vi "GaussianFit1D.vi"(0 "Cut":dbl[](graph)=[201.0, 170.0, 133.0, 114.0, 97.0, 133.0, 100.0, 5.0, 49.0, 50.0, 23.0, -22.0, -18.0, 16.0, 32.0, 1.0, -40.0, -42.0, -16.0, 11.0, -45.0, 12.0, -44.0, 20.0, -75.0, -48.0, 7.0, -12.0, -59.0, -11.0, -91.0, -34.0, -8.0, 3.0, -81.0, -7.0, -61.0, -16.0, -12.0, -87.0, -53.0, -14.0, -17.0, -15.0, -2.0, -87.0, -43.0, -62.0, -21.0, -22.0, -84.0, 12.0, -74.0, -15.0, -65.0, -10.0, 23.0, -6.0, 151.0, 386.0, 1054.0, 2361.0, 4328.0, 5745.0, 7056.0, 6029.0, 3889.0, 2158.0, 764.0, 178.0, -14.0, -30.0, 42.0, 60.0, -25.0, 8.0, -41.0, 24.0, -82.0, -31.0, 3.0, -2.0, 44.0, -60.0, -18.0, 0.0, 33.0, 26.0, -27.0, -29.0, -16.0, 19.0, 14.0, -10.0, -36.0, -47.0, -663.0, -28.0, -32.0, -7.0]) -> (1 "Sigma":dbl format="%.2f", 2 "x":dbl format="%.2f")   [LabVIEW 2009]
uses:
  <vilib>/gmath/NI_Gmath.lvlib
  <vilib>/Analysis/NI_AALBase.lvlib
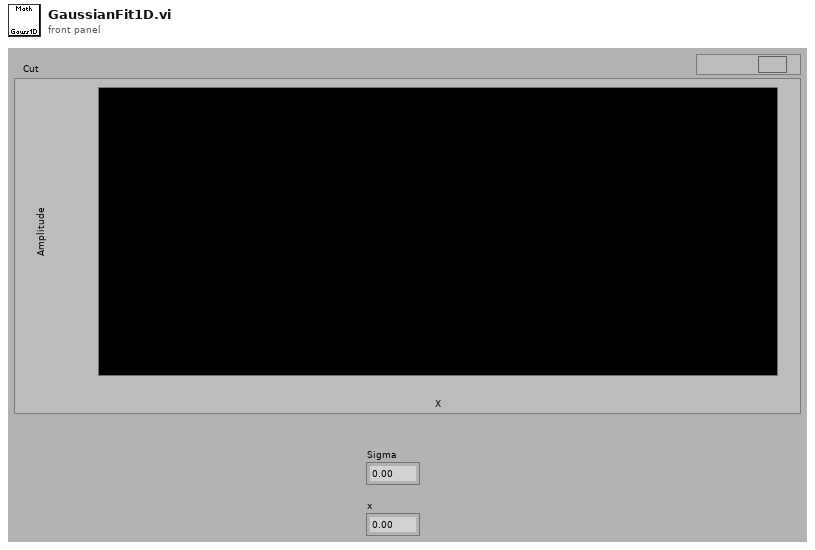
[diagram p1: front panel]
types:
  T1 = cluster{"model":string, "Parameters":string[], "x":string}
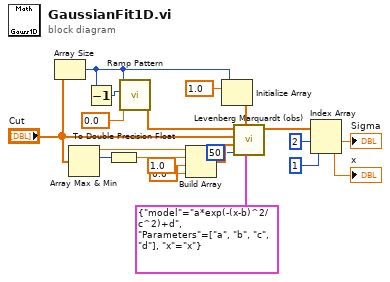
[diagram p0: block diagram]
diagram:
  n1 = Array Size(array="Cut") -> (size(s)=w15:i32)
  n2 = Array Max & Min(array="Cut") -> (max value=w12:dbl, max index (indices)=w10:i32)  [unwired: 2 out]
  n3 = Decrement(x=w15) -> (x-1=w19:i32)
  n4 = To Double Precision Float(number=w10) -> (double precision float=w9:dbl)
  n5 = call <vilib>:"Ramp Pattern.vi"("start"=0.0, "end"=w19, "samples"=w15) -> ("Ramp Pattern"=w18:dbl[])  [unwired: 7 in, 1 out]
  n6 = Build Array(w12, w9, 1.0 ("élément"), 0.0 ("élément")) -> (w11:dbl[])
  n7 = Initialize Array(1.0 ("élément"), w15) -> (w16:dbl[])
  n8 = call <vilib>:"Levenberg Marquardt (obs).vi"("model description"=T1 {"model"="a*exp(-(x-b)^2/c^2)+d", "Parameters"=["a", "b", "c", "d"], "x"="x"}, "Standard Deviation"=w16, "max iteration"=50, "Initial Guess Coefficient"=w11, "Y"="Cut", "X"=w18) -> ("Best Fit Coefficients"=w7:dbl[])  [unwired: 5 out]
  n9 = Index Array(array=w7, index #1=2 ("indice"), index #2=1 ("indice")) -> (element #1=→"Sigma":dbl, element #2=→"x":dbl)
